vi "write general keywords.vi"(8 "error in (no error)":errorcluster, 11 "Save Image in":refnum<class "Save Image.lvclass">) -> (0 "error out":errorcluster, 3 "Save Image out":refnum<class "Save Image.lvclass">)   [LabVIEW 2018, in "Save Image.lvclass"]
uses:
  Save Image.lvclass
  Save Image.lvclass/Save Image.ctl
  Channel/Channel.lvclass/Channel.ctl
  Simulated_CCD_Camera/Simulated Camera.lvclass
  Channel/Channel.lvclass
panel:
  in  "Channel information":T1
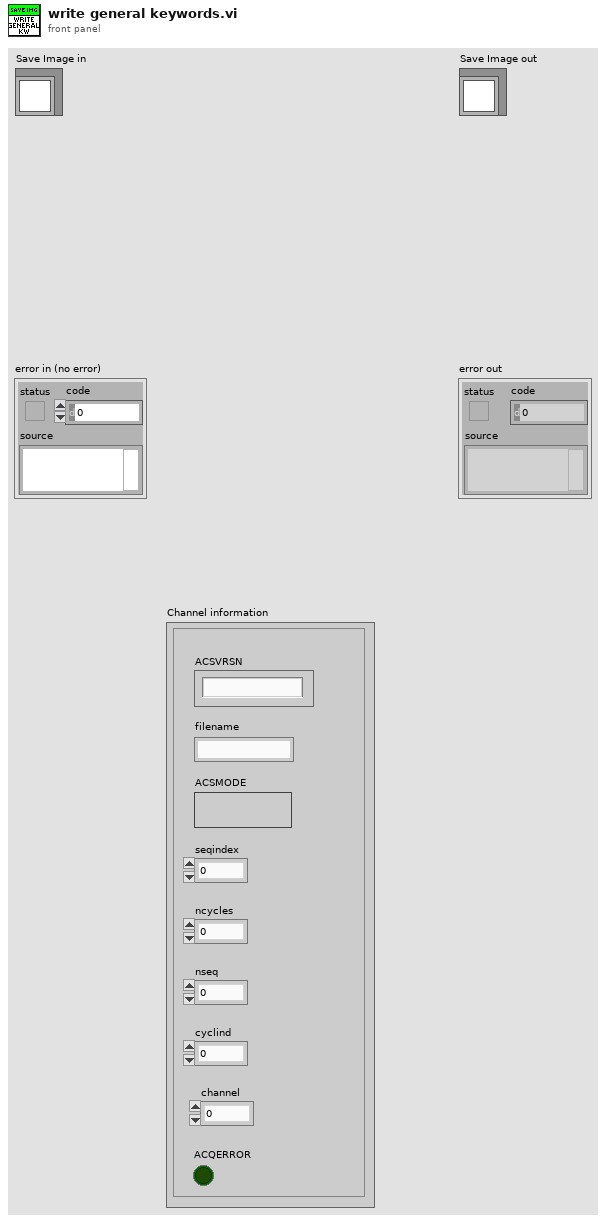
[diagram p1: front panel]
types:
  T1 = cluster{"ACSVRSN":string, "ACSMODE":bool, "filename":string, "seqindex":u16, "ncycles":u16, "nseq":u16, "cyclind":u16, "channel":u16, "ACQERROR":bool}
  T2 = cluster{"Image path":path, "Remote IP":string, "Channel":u8, "ACS mode":u16, "Communication":u16}
  T3 = cluster{"CYCLES_DONE":u16, "LAST_IMAGE_NAME":string, "USED_DISK_SPACE":u16, "FRAMES_DONE":u16, "CCD_STATUS":string, "CURRENT_TEMPERATURE":i16, "TEMPERATURE_STATUS":string, "FRAME_EXPOSURE_TIME":sgl, "ERROR":bool, "SERIAL_NUMBER":u16, "ACQUIRING":bool, "IMAGE_INDEX":u32, "SEQS_DONE":u16}
  T4 = cluster{"COOLER_POWER_STATUS":u16, "TEMP":i32, "EXPTIME":dbl, "#FRAMES":u32, "#CYCLES":u32, "#SEQS":u32, "WAVEPLATE_POS":u16}
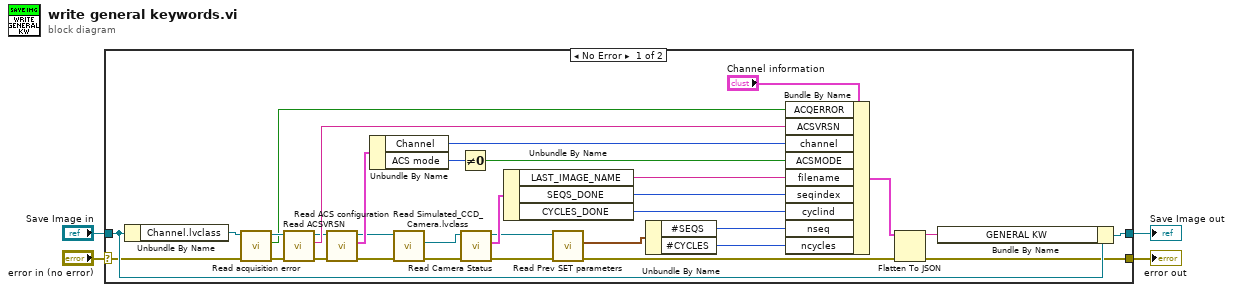
[diagram p0: block diagram]
diagram:
  n1 = case shown="No Error" "error in (no error)" {
    selector: "error in (no error)" -> [w6 w38]
    tunnel: [w18 w38] -> w3
    tunnel: [w15 w37] -> w1
    tunnel: "Save Image in" -> [w20 w37]
    frame No Error {
      n2 = Unbundle By Name(w20) -> ("Channel.lvclass"=w9:refnum<class "Channel.lvclass">)
      n3 = call-dynamic "Read acquisition error.vi"("error in (no error)"=w6, "Channel in"=w9) -> ("error out"=w7:errorcluster, "acquisition error"=w5:bool, "Channel out"=w8:refnum<class "Channel.lvclass">)  [unwired: 7 in]
      n4 = call "Read ACSVRSN.vi"("error in (no error)"=w7, "Channel in"=w8) -> ("error out"=w11:errorcluster, "ACSVRSN"=w35:string, "Channel out"=w12:refnum<class "Channel.lvclass">)  [unwired: 7 in]
      n5 = call-dynamic "Read ACS configuration.vi"("error in (no error)"=w11, "Channel in"=w12) -> ("error out"=w34:errorcluster, "acs init configuration"=w36:T2, "Channel out"=w33:refnum<class "Channel.lvclass">)  [unwired: 7 in]
      n6 = Unbundle By Name(w36) -> ("Channel"=w10:u8, "ACS mode"=w13:u16)
      n7 = call "Read Simulated_CCD_Camera.lvclass.vi"("error in (no error)"=w34, "Channel in"=w33) -> ("error out"=w31:errorcluster, "Simulated_CCD_Camera.lvclass"=w32:refnum<class "Simulated Camera.lvclass">)  [unwired: 7 in, 1 out]
      n8 = Not Equal To 0?(x=w13) -> (x != 0?=w14:bool)
      n9 = call "Read Camera Status.vi"("error in (no error)"=w31, "CCDCamera in"=w32) -> ("error out"=w30:errorcluster, "Camera Status"=w29:T3, "CCDCamera out"=w22:refnum<class "Simulated Camera.lvclass">)  [unwired: 7 in]
      n10 = Unbundle By Name(w29) -> ("LAST_IMAGE_NAME"=w28:string, "SEQS_DONE"=w27:u16, "CYCLES_DONE"=w26:u16)
      n11 = call-dynamic "Read Prev SET parameters.vi"("error in (no error)"=w30, "Simulated_CCD_Camera in"=w22) -> ("error out"=w19:errorcluster, "Prev SET parameters"=w25:T4)  [unwired: 7 in, 1 out]
      n12 = Unbundle By Name(w25) -> ("#SEQS"=w24:u32, "#CYCLES"=w23:u32)
      n13 = Bundle By Name(cluster="Channel information", "ACQERROR"=w5, "ACSVRSN"=w35, "channel"=w10, "ACSMODE"=w14, "filename"=w28, "seqindex"=w27, "cyclind"=w26, "nseq"=w24, "ncycles"=w23) -> (w16:T1)
      n14 = Flatten To JSON(anything=w16, error in (no error)=w19) -> (JSON string=w17:string, 11:w18:errorcluster)  [unwired: 1 in]
      n15 = Bundle By Name(cluster=w20, "GENERAL KW"=w17) -> (w15:refnum<class "Save Image.lvclass">)
    }
    frame Error {
    }
  }
  "error out" <- w3
  "Save Image out" <- w1
